vi "DataLog Log String.vi"(0 "tag":string, 5 "string":string, 7 "time":dbl format="%<%H:%M:%S%2u\n%Y/%m/%d>T", 9 "database (current)":string, 11 "error in (no error)":errorcluster) -> (15 "error out":errorcluster)   [LabVIEW 2012]
doc: "Normally you should use \"Write String\" to log a string to a tag. This subVI should NOT be used unless you must be able to write a string to a database that is not necessarily live (for which datalogging might not be active). This is intended mainly for logging errors and warnings such that they show up in the database even when they occur before the database has gone live.\n\nWhen the current database is live, the normal buffered logging mechanism is used. Otherwise the string tag log is directly appended to without in-memory buffering. This subVI is smart enough to keep on functioning when the system has only partially initialised towards or cleaned up from a live logging state: when the database is live, it first tries buffered string writing and, when that fails, it attempts the direct approach."
uses:
  typedefs/t_DataLog Databases Methods.ctl
  typedefs/t_DataLog Tag Info List Methods.ctl
  typedefs/t_Datalog Datebase Modes.ctl
  typedefs/clusters/t_DataLog Point.ctl
  glb_DataLog MCVD.vi
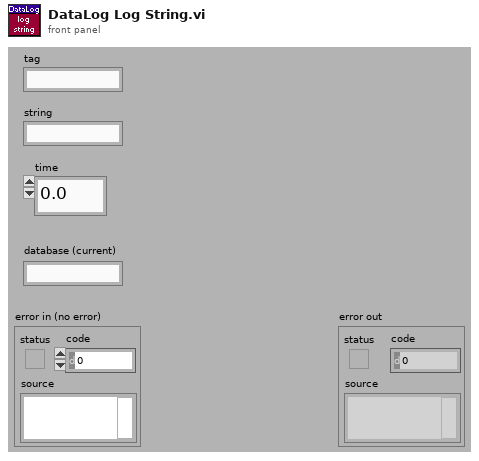
[diagram p1: front panel]
types:
  T1 = typedef "t_DataLog Databases Methods.ctl" = enum16{"initialize", "get ref", "get names", "cleanup"}
  T2 = typedef "t_DataLog Database Info Pane.ctl" = refnum<vi>
  T3 = typedef "t_DataLog Tag Info List Methods.ctl" = enum16{"initialize", "create", "create empty", "rename", "delete", "test tag", "get", "get by name", "get default", "get list", "get path", "get subsets", "set subsets", "set config", "set capacity", "#tags", "go live", "set unlocked", "set mirrored"}
  T4 = typedef "t_DataLog Point.ctl" = cluster{"time":dbl, "value":dbl}
  T5 = typedef "t_Datalog Datebase Modes.ctl" = enum16{"locked", "unlocked", "live", "mirrored"}
  T6 = typedef "t_DataLog Tag Config.ctl" = cluster{"name":string, "unit":string, "temporal":T7, "value":T8, "index":i32, "capacity":i32, "is meta?":bool, "mincapacity":i32, "deadband":dbl, "limit delay":dbl, "format":T9, "precision":u8, "undefine":bool, "update":bool, "update period":u16, "expression":string, "description":string, "logging algorithm":T10, "logging parameters":dbl[]}
  T7 = typedef "t_DataLog Temporal Types.ctl" = enum16{"set&hold", "sample", "event"}
  T8 = typedef "t_DataLog Value Types.ctl" = enum16{"number", "string"}
  T9 = typedef "t_DataLog Numerical Format.ctl" = enum8{"fractional", "exponential", "engineering"}
  T10 = typedef "t_DataLog Logging Algorithms.ctl" = enum16{"nothing", "changes", "everything", "every Nth", "time threshold", "value threshold + prior", "t or v threshold", "t or v threshold + prior"}
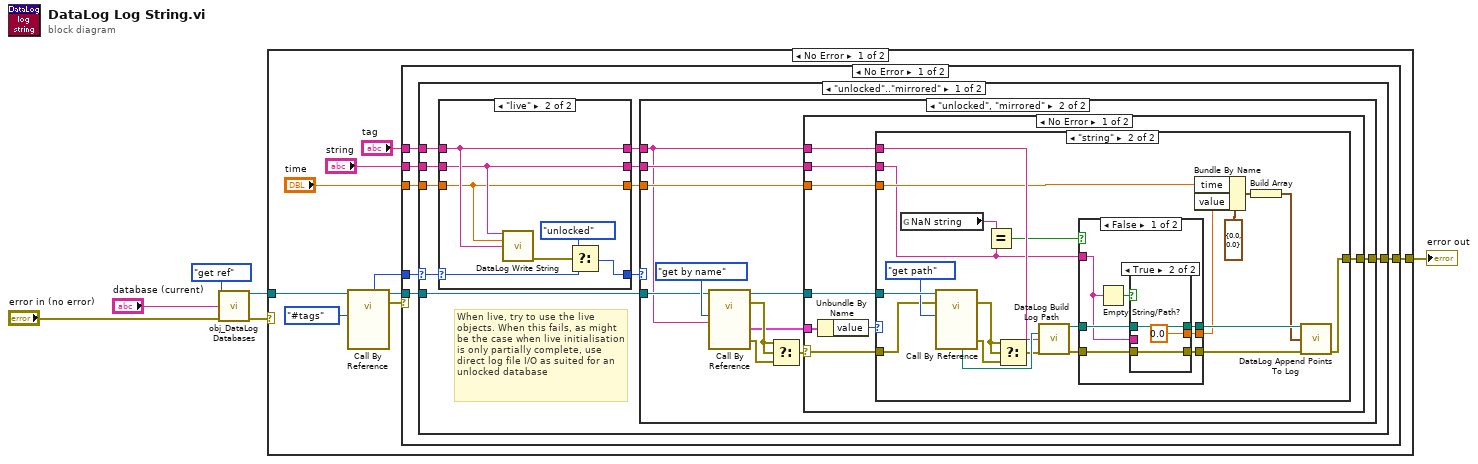
[diagram p0: block diagram]
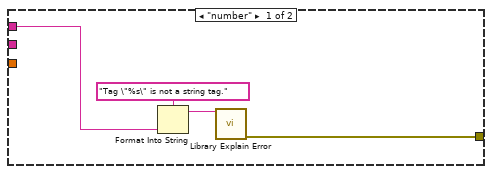
[diagram p3: hidden frame]
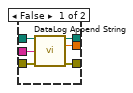
[diagram p4: hidden frame]
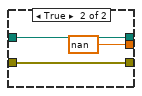
[diagram p5: hidden frame]
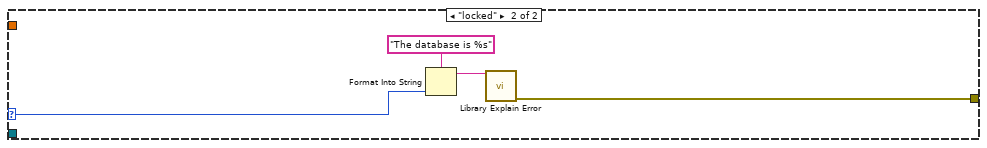
[diagram p8: hidden frame]
diagram:
  n1 = call "obj_DataLog Databases.vi"("method"=t_DataLog_Databases_Methods."get ref", "database (current)"="database (current)", "error in (no error)"="error in (no error)") -> ("database ref"=w4:T2, "error out"=w5:errorcluster)  [unwired: 10 in, 1 out]
  n2 = case shown="No Error" w5 {
    selector: w5 -> [_ w112]
    tunnel: w4 -> [w15 _]
    tunnel: [w11 w112] -> w1
    frame No Error {
      n3 = call-by-ref "?"(reference=w15, "method"=t_DataLog_Tag_Info_List_Methods."#tags") -> (reference out=w12:T2, error out=w10:errorcluster, "mode"=w13:T5)  [unwired: 9 in, 6 out]
      n4 = case shown="No Error" w10 {
        selector: w10 -> [_ w111]
        tunnel: w13 -> [w21 _]
        tunnel: w12 -> [w20 _]
        tunnel: [w19 w111] -> w11
        tunnel: "tag" -> [w18 _]
        tunnel: "string" -> [w17 _]
        tunnel: "time" -> [w16 _]
        frame No Error {
          n5 = case shown="\"unlocked\"..\"mirrored\"" w21 {
            selector: w21 -> [w28 w109]
            tunnel: w20 -> [w23 _]
            tunnel: [w22 w110] -> w19
            tunnel: w18 -> [w29 _]
            tunnel: w17 -> [w31 _]
            tunnel: w16 -> [w30 _]
            frame "unlocked".."mirrored" {
              # "When live, try to use the live objects. When this fails, as might be the case when live initialisation is only partially complete, use direct log file I/O as suited for an unlocked database"
              n6 = case shown="\"live\"" w28 {
                selector: w28 -> [w96 w106]
                tunnel: w31 -> [w98 w101]
                tunnel: w30 -> [w97 w100]
                tunnel: w29 -> [w99 w102]
                tunnel: [w99 w102] -> w24
                tunnel: [w98 w101] -> w25
                tunnel: [w97 w100] -> w26
                tunnel: [w96 w104] -> w27
                frame Default {
                }
                frame "live" {
                  n7 = call "DataLog Write String.vi"("string"=w101, "time (current)"=w100, "tag"=w102) -> ("error out"=w103:errorcluster)  [unwired: 11 in, 1 out]
                  n8 = Select(t=t_Datalog_Datebase_Modes."unlocked" ("mode"), s=w103, f=w106) -> (s? t:f=w104:T5)
                }
              }
              n9 = case shown="\"unlocked\", \"mirrored\"" w27 {
                tunnel: w25 -> [_ w36]
                tunnel: w26 -> [_ w35]
                tunnel: w24 -> [_ w32]
                tunnel: w23 -> [_ w38]
                tunnel: [_ w33] -> w22
                frame Default {
                }
                frame "unlocked", "mirrored" {
                  n10 = call-by-ref "?"(reference=w38, "method"=t_DataLog_Tag_Info_List_Methods."get by name", "tag or base tag"=w32) -> (reference out=w42:T2, error out=w41:errorcluster, "tag config out"=w37:T6, 15:"error out"=w40:errorcluster)  [unwired: 8 in, 5 out]
                  n11 = Select(t=w41, s=w41, f=w40) -> (s? t:f=w34:errorcluster)
                  n12 = case shown="No Error" w34 {
                    selector: w34 -> [w48 w95]
                    tunnel: w42 -> [w50 _]
                    tunnel: w37 -> [w49 _]
                    tunnel: w36 -> [w44 _]
                    tunnel: w35 -> [w43 _]
                    tunnel: [w46 w95] -> w33
                    tunnel: w32 -> [w45 _]
                    frame No Error {
                      n13 = Unbundle By Name(w49) -> ("value"=w47:T8)
                      n14 = case shown="\"string\"" w47 {
                        tunnel: w50 -> [_ w73]
                        tunnel: w48 -> [_ w69]
                        tunnel: [w52 w60] -> w46
                        tunnel: w45 -> [w51 w68]
                        tunnel: w44 -> [_ w55]
                        tunnel: w43 -> [_ w62]
                        frame "number" {
                          n15 = Format Into String(format string="Tag \"%s\" is not a string tag.", w51) -> (resulting string=w53:string)  [unwired: 2 in, 1 out]
                          n16 = call "Library Explain Error.vi"("explanation prefix (none)"=w53) -> ("explained error"=w52:errorcluster)  [unwired: 14 in]
                        }
                        frame "string" {
                          n17 = global read "glb_DataLog MCVD.vi" "NaN string"() -> (w57:string)
                          n18 = call-by-ref "?"(reference=w73, error in=w69, "method"=t_DataLog_Tag_Info_List_Methods."get path") -> (error out=w70:errorcluster, "path"=w75:path, 15:"error out"=w71:errorcluster)  [unwired: 8 in, 6 out]
                          n19 = Equal?(x=w57, y=w55) -> (x = y?=w56:bool)
                          n20 = Select(t=w70, s=w70, f=w71) -> (s? t:f=w74:errorcluster)
                          n21 = call "DataLog Build Log Path.vi"("database path"=w75, "tag"=w68, "error in (no error)"=w74) -> ("tag log directory"=w66:path, "error out"=w67:errorcluster)  [unwired: 11 in]
                          n22 = case shown="False" w56 {
                            tunnel: w67 -> [w82 w94]
                            tunnel: w66 -> [w81 w93]
                            tunnel: [w80 w94] -> w65
                            tunnel: [w79 w93] -> w64
                            tunnel: [w78 nan ("offset")] -> w61
                            tunnel: w55 -> [w76 _]
                            frame False {
                              n23 = Empty String/Path?(string/path=w76) -> (empty?=w77:bool)
                              n24 = case shown="True" w77 {
                                tunnel: w82 -> [w88 w90]
                                tunnel: w81 -> [w87 w91]
                                tunnel: [w86 w90] -> w80
                                tunnel: [w85 w91] -> w79
                                tunnel: [w84 0.0 ("offset")] -> w78
                                tunnel: w76 -> [w83 _]
                                frame False {
                                n25 = call "DataLog Append String.vi"("tag log directory"=w87, "string"=w83, "error in (no error)"=w88) -> ("dup tag log directory"=w85:path, "offset"=w84:dbl, "error out"=w86:errorcluster)  [unwired: 9 in, 1 out]
                                }
                                frame True {
                                }
                              }
                            }
                            frame True {
                            }
                          }
                          n26 = Bundle By Name(cluster=T4 {"time"=0.0, "value"=0.0} ("point"), "time"=w62, "value"=w61) -> (w59:T4)
                          n27 = Build Array(w59) -> (w58:T4[])
                          n28 = call "DataLog Append Points To Log.vi"("tag log directory"=w64, "points"=w58, "error in (no error)"=w65) -> ("error out"=w60:errorcluster)  [unwired: 11 in, 1 out]
                        }
                      }
                    }
                    frame Error {
                    }
                  }
                }
              }
            }
            frame "locked" {
              n29 = Format Into String(format string="The database is %s", w109) -> (resulting string=w108:string)  [unwired: 2 in, 1 out]
              n30 = call "Library Explain Error.vi"("explanation prefix (none)"=w108) -> ("explained error"=w110:errorcluster)  [unwired: 14 in]
            }
          }
        }
        frame Error {
        }
      }
    }
    frame Error {
    }
  }
  "error out" <- w1
